vi "getStringRepresentation.vi"(11 "Delimiter in":refnum<class "Delimiter.lvclass">) -> (2 "String representation":string, 3 "Delimiter out":refnum<class "Delimiter.lvclass">)   [LabVIEW 2014, in "Delimiter.lvclass"]
uses:
  Delimiter.lvclass
  Delimiter.lvclass/Delimiter.ctl
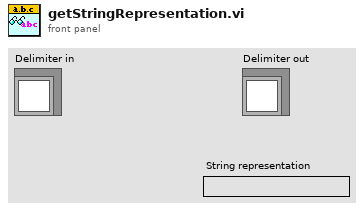
[diagram p1: front panel]
types:
  T1 = typedef "Delimiter.lvclass/Delimiters List.ctl" = enum16{"Default", "dot (.)", "colon (:)", "double-colon (::)", "semi-colon (;)", "underscore (_)", "double underscore (__)", "dash (-)", "double dash (--)", "backslash (\\)", "vertical bar (|)", "forward slash (/)", "chevron (>)", "double-chevron (>>)", "arrow (->)", "comma (,)", "arobas (@)", "ampersand (&)", "other"}
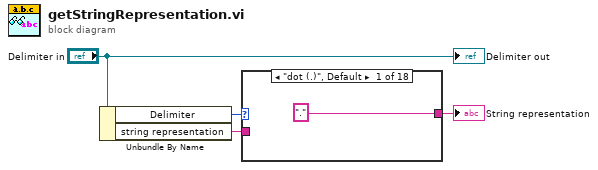
[diagram p0: block diagram]
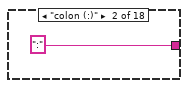
[diagram p2: hidden frame]
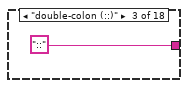
[diagram p3: hidden frame]
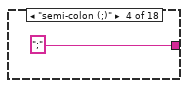
[diagram p4: hidden frame]
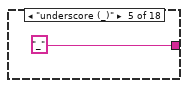
[diagram p5: hidden frame]
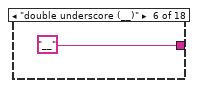
[diagram p6: hidden frame]
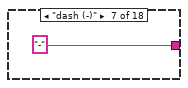
[diagram p7: hidden frame]
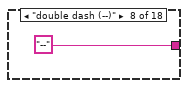
[diagram p8: hidden frame]
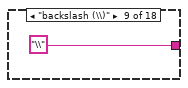
[diagram p9: hidden frame]
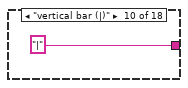
[diagram p10: hidden frame]
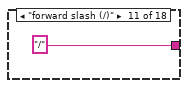
[diagram p11: hidden frame]
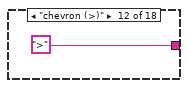
[diagram p12: hidden frame]
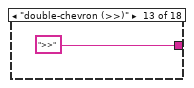
[diagram p13: hidden frame]
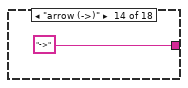
[diagram p14: hidden frame]
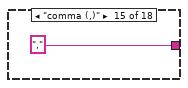
[diagram p15: hidden frame]
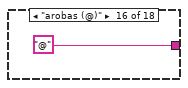
[diagram p16: hidden frame]
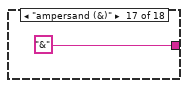
[diagram p17: hidden frame]
diagram:
  n1 = Unbundle By Name("Delimiter in") -> ("Delimiter"=w2:T1, "string representation"=w1:string)
  n2 = case shown="\"dot (.)\", Default" w2 {
    tunnel: ["." ":" "::" ";" "_" "__" "-" "--" "\\" "|" "/" ">" ">>" "->" "," "@" "&" w22] -> w4
    tunnel: w1 -> [_ _ _ _ _ _ _ _ _ _ _ _ _ _ _ _ _ w22]
    frame "dot (.)", Default {
    }
    frame "colon (:)" {
    }
    frame "double-colon (::)" {
    }
    frame "semi-colon (;)" {
    }
    frame "underscore (_)" {
    }
    frame "double underscore (__)" {
    }
    frame "dash (-)" {
    }
    frame "double dash (--)" {
    }
    frame "backslash (\\)" {
    }
    frame "vertical bar (|)" {
    }
    frame "forward slash (/)" {
    }
    frame "chevron (>)" {
    }
    frame "double-chevron (>>)" {
    }
    frame "arrow (->)" {
    }
    frame "comma (,)" {
    }
    frame "arobas (@)" {
    }
    frame "ampersand (&)" {
    }
    frame "other" {
    }
  }
  "String representation" <- w4
  "Delimiter out" <- "Delimiter in"
